vi "Sub Initialize.vi"(8 "error in (no error)":errorcluster, 11 "Timer in":refnum<class "Timer.lvclass">) -> (0 "error out":errorcluster, 2 "Initialize Result":refnum<class "Acquired Result.lvclass">, 3 "Timer out":refnum<class "Timer.lvclass">)   [LabVIEW 2019, in "Timer.lvclass"]
uses:
  Timer.lvclass
  C:/GitHub/LabActor/Worker/Worker.lvclass
  NHMFL_Core/Libraries/Instruments/Results/Acquired Result/Acquired Result.lvclass
  NHMFL_Core/Libraries/Instruments/Results/Start Stream Result/Start Stream Result.lvclass
  C:/GitHub/NHMFL_Core/Libraries/Instruments/Results/Acquired Result/Acquired Result.lvclass
  Timer.lvclass/Timer.ctl
  Worker/Worker.lvclass/Worker.ctl
  NHMFL_Core/Libraries/Instruments/Results/Start Stream Result/Start Stream Result.lvclass/Start Stream Result.ctl
  NHMFL_Core/Libraries/Instruments/Results/Acquired Result/Acquired Result.lvclass/Acquired Result.ctl
  Write Start time.vi
  Write Latest time.vi
  Write First call.vi
  Write Delay active.vi
  Worker/Read Cycle period.vi
  NHMFL_Core/Libraries/Instruments/Results/Start Stream Result/Write dt.vi
  NHMFL_Core/Libraries/Instruments/Results/Acquired Result/Write Channels.vi
  NHMFL_Core/Libraries/Instruments/Results/Acquired Result/Write Group.vi
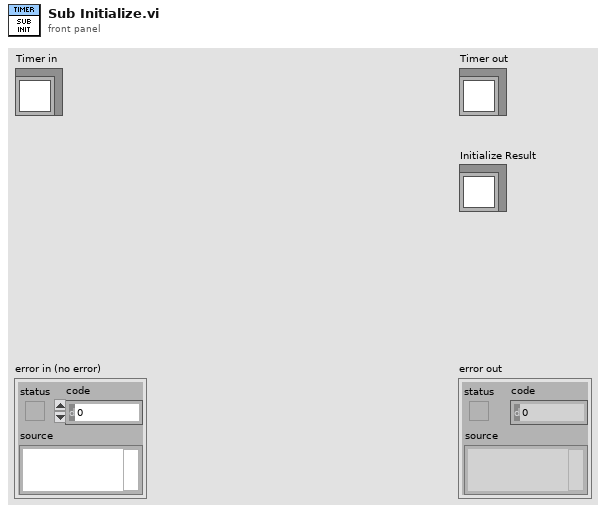
[diagram p1: front panel]
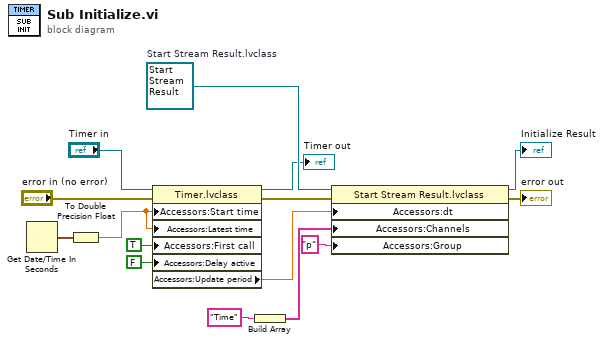
[diagram p0: block diagram]
diagram:
  w14 = refnum<class "Start Stream Result.lvclass"> refnum  # Start Stream Result.lvclass
  n1 = Get Date/Time In Seconds() -> (seconds since 1Jan1904=w15:timestamp)
  n2 = To Double Precision Float(number=w15) -> (double precision float=w1:dbl)
  n3 = property class="Timer.lvclass"(reference="Timer in", error in="error in (no error)", "Accessors:Start time"=w1, "Accessors:Latest time"=w1, "Accessors:First call"=TRUE ("First call"), "Accessors:Delay active"=FALSE ("Delay active")) -> (reference out=→"Timer out":refnum<class "Timer.lvclass">, error out=w12:errorcluster, "Accessors:Update period"=w2:dbl)
  n4 = Build Array("Time") -> (w3:string[])
  n5 = property class="Start Stream Result.lvclass"(reference=w14, error in=w12, "Accessors:dt"=w2, "Accessors:Channels"=w3, "Accessors:Group"="p" ("Group")) -> (reference out=→"Initialize Result":refnum<class "Start Stream Result.lvclass">, error out=→"error out":errorcluster)
